vi "coord.vi"(7 "error in":errorcluster) -> (27 "error out":errorcluster)   [LabVIEW 2019]
uses:
  <vilib>/vision/Pattern Matching.llb/IMAQ Pattern Match Advanced Options.ctl
  <vilib>/vision/NI_Vision_Development_Module.lvlib
panel:
  in  "selected path":path
  out "ROI Descriptor out":T1 {"Contours"."Type" items=["No Selection", "Point", "Line", "Rectangle", "Oval", "Polygon", "Freehand Region", "Annulus", "Unused2", "Unused3", "Broken Line", "Freehand Line", "Rotated Rectangle"]}
  out "Image Out":T2(plugin-control)
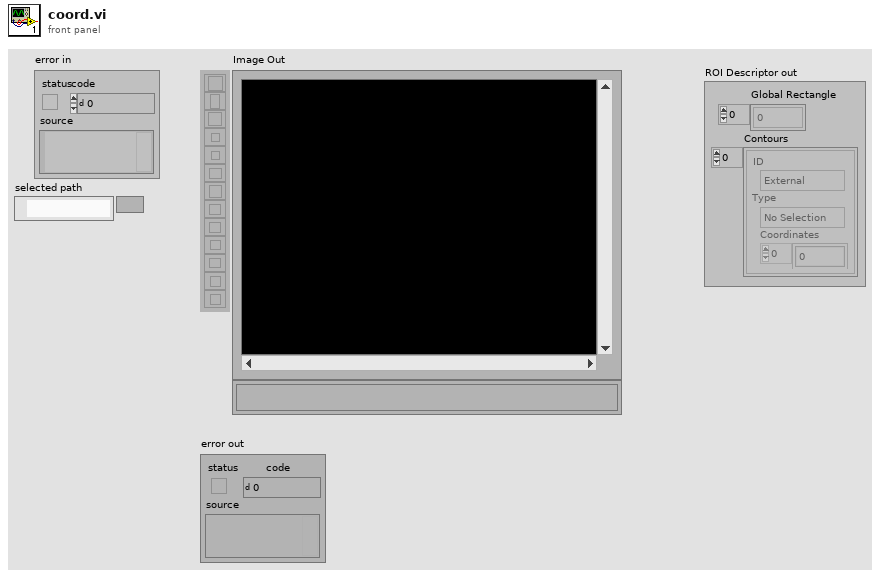
[diagram p1: front panel]
types:
  T1 = typedef "ROI Descriptor" = cluster{"Global Rectangle":i32[], "Contours":cluster{"ID":enum32{"External", "Internal"}, "Type":u32, "Coordinates":i32[]}[]}
  T2 = typedef "IMAQ Image.ctl" = refnum<image>
  T3 = cluster{"Global Rectangle":i32[], "Contours":cluster{"ID":enum32{"External", "Internal"}, "Type":u32, "Coordinates":i32[]}[]}
  T4 = cluster{"Origin":cluster{"X":sgl, "Y":sgl}, "Angle (deg)":sgl, "Axis Reference":u32}
  T5 = enum16{"Reset", "Update Coordinate System", "Get Coordinate System"}
  T6 = enum16{"Horizontal Motion", "Vertical Motion", "Horizontal and Vertical Motion", "Horizontal, Vertical and Angular Motion"}
  T7 = typedef "IMAQ Pattern Match Advanced Options.ctl" = u16
  T8 = cluster{"Number of Matches Requested":i32, "Minimum Match Score":sgl, "Angle Ranges":cluster{"Start Angle":sgl, "End Angle":sgl}[]}
  T9 = typedef "Image Type" = u32
  T10 = cluster{"Position":cluster{"x":sgl, "y":sgl}, "Angle":sgl, "Scale":sgl, "Score":sgl, "Bounding Box":cluster{"x":sgl, "y":sgl}[]}[]
  T11 = typedef "IMAQ Coordinate System" = cluster{"Reference System":cluster{"Origin":cluster{"X":sgl, "Y":sgl}, "Angle (deg)":sgl, "Axis Reference":u32}, "Measurement System":cluster{"Origin":cluster{"X":sgl, "Y":sgl}, "Angle (deg)":sgl, "Axis Reference":u32}}
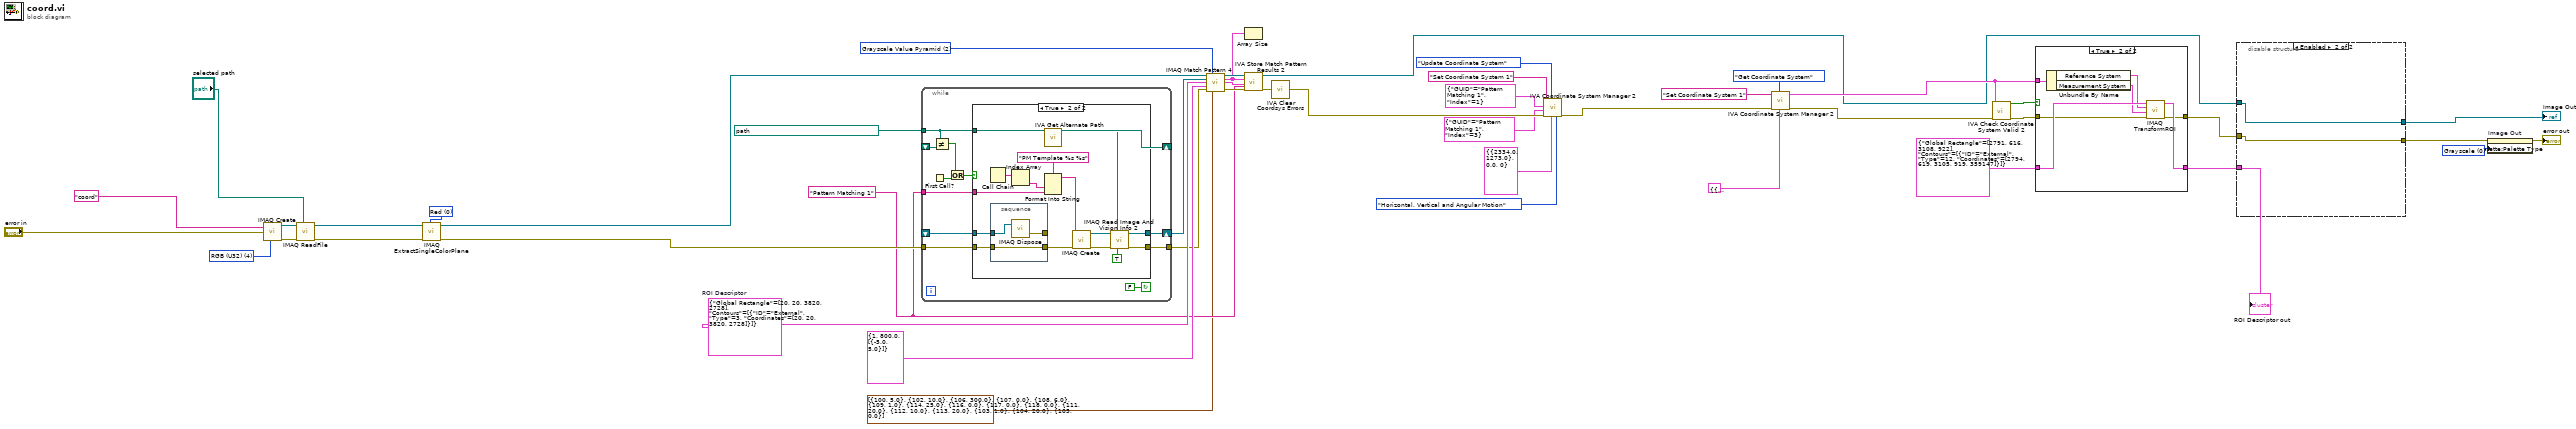
[diagram p0: block diagram]
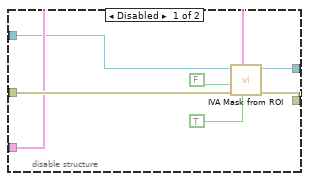
[diagram p2: hidden frame]
diagram:
  w3 = u32 0 items=["Grayscale", "Binary", "Gradient", "Rainbow", "Temperature", "User Defined", "Binary 16 Bit", "Gradient 16 Bit", "Rainbow 16 Bit", "Temperature 16 Bit", "User Defined 16 Bit"] ("Palette Type")
  w35 = 2 items=["All", "Low Discrepancy Sampling", "Grayscale Value Pyramid", "Gradients Pyramid"] ("Algorithm")
  w32 = "Pattern Matching 1" ("Step Name")
  w34 = T3 {"Global Rectangle"=[20, 20, 3820, 2728], "Contours"=[{"ID"=enum."External", "Type"=3, "Coordinates"=[20, 20, 3820, 2728]}]}  # ROI Descriptor
  w42 = 0 items=["Red", "Green", "Blue", "Hue", "Saturation", "Luminance", "Value", "Intensity"] ("Color Plane")
  w43 = T9 4 items=["Grayscale (U8)", "Grayscale (I16)", "Grayscale (SGL)", "Complex (CSG)", "RGB (U32)", "HSL (U32)", "RGB (U64)", "Grayscale (U16)"] ("Image Type")
  n1 = call "IMAQ Create"("Image Name"="coord", "Image Type"=w43, "error in (no error)"="error in") -> ("New Image"=w46:T2, "error out"=w45:errorcluster)  [unwired: 1 in, 1 out]
  n2 = call "IMAQ ReadFile"("File Path"="selected path", "error in (no error)"=w45, "Image"=w46) -> ("error out"=w47:errorcluster, "Image Out"=w41:T2)  [unwired: 2 in, 5 out]
  n3 = call "IMAQ ExtractSingleColorPlane"("Color Plane"=w42, "error in (no error)"=w47, "Image Src"=w41) -> ("error out"=w40:errorcluster, "Image Dst Out"=w38:T2)  [unwired: 1 in, 6 out]
  n4 = while {
    shift-right: [w58] -> w29
    shift-left: _ -> [w57]
    tunnel: [w55] -> w28
    tunnel: w40 -> [w54]
    tunnel: path "D:/vicomm case/為生 AI/AI Picture/11.png" ("Template File Path") -> [w51]
    tunnel: w32 -> [w53]
    shift-right: [w51] -> _
    shift-left: _ -> [w52]
    stop <- FALSE continue-if-true
    n5 = First Call?() -> (First Call?: T/F=w50:bool)
    n6 = Not Equal?(x=w51, y=w52) -> (x != y?=w49:bool)
    n7 = Or(x=w49, y=w50) -> (x .or. y?=w48:bool)
    n8 = case shown="True" w48 {
      tunnel: [w60 w65] -> w58
      tunnel: w57 -> [w60 w69]
      tunnel: [w59 w66] -> w55
      tunnel: w54 -> [w59 w68]
      tunnel: w51 -> [_ w70]
      tunnel: w53 -> [_ w71]
      frame False {
      }
      frame True {
        n9 = Call Chain() -> (call chain=w73:string[])
        n10 = stacked-sequence {
          tunnel: w69 -> [w78]
          tunnel: w68 -> [w77]
          tunnel: [w77] -> w62
          tunnel: [w76] -> _
          frame #0 {
            n11 = call "IMAQ Dispose"("Image"=w78) -> ("error out"=w76:errorcluster)  [unwired: 2 in, 3 out]
          }
        }
        n12 = Index Array(array=w73) -> (element=w72:string)  [unwired: 1 in]
        n13 = call <vilib>:"IVA Get Alternate Path.vi"("Path In"=w70) -> ("Path Out"=w67:path)  [unwired: 10 out]
        n14 = Format Into String(format string="PM Template %s %s" ("Image Name"), w72, w71) -> (resulting string=w75:string)  [unwired: 2 in, 1 out]
        n15 = call "IMAQ Create"("Image Name"=w75, "error in (no error)"=w62) -> ("New Image"=w64:T2, "error out"=w63:errorcluster)  [unwired: 2 in, 1 out]
        n16 = call "IMAQ Read Image And Vision Info 2"("Use File Path Image Type"=TRUE, "File Path"=w67, "error in (no error)"=w63, "Image"=w64) -> ("error out"=w66:errorcluster, "Image Out"=w65:T2)  [unwired: 5 in, 1 out]
      }
    }
  }
  n17 = call "IMAQ Match Pattern 4"("Image"=w38, "Algorithm"=w35, "Template Image"=w29, "ROI Descriptor"=w34, "Parameters"=T8 {"Number of Matches Requested"=1, "Minimum Match Score"=800.0, "Angle Ranges"=[{"Start Angle"=-5.0, "End Angle"=5.0}]}, "error in (no error)"=w28, "Advanced Options"=cluster{"Item":T7, "Value":dbl}[] [{"Item"=100, "Value"=5.0}, {"Item"=102, "Value"=10.0}, {"Item"=106, "Value"=300.0}, {"Item"=107, "Value"=0.0}, {"Item"=108, "Value"=6.0}, {"Item"=109, "Value"=1.0}, {"Item"=114, "Value"=25.0}, {"Item"=116, "Value"=0.0}, {"Item"=117, "Value"=0.0}, {"Item"=118, "Value"=0.0}, {"Item"=111, "Value"=20.0}, {"Item"=112, "Value"=10.0}, {"Item"=113, "Value"=20.0}, {"Item"=103, "Value"=1.0}, {"Item"=104, "Value"=20.0}, {"Item"=105, "Value"=0.0}]) -> ("Image (duplicate)"=w36:T2, "Matches (pixel)"=w31:T10, "Matches (real-world)"=w30:T10, "error out"=w37:errorcluster)  [unwired: 4 in, 1 out]
  n18 = Array Size(array=w31) -> ()  [unwired: 1 out]
  n19 = call <vilib>:"IVA Store Match Pattern Results 2.vi"("Step Name"=w32, "error in (no error)"=w37, "Matches (real-world)"=w30, "Matches (pixel)"=w31, "Image in"=w36) -> ("error out"=w27:errorcluster, "Image dup"=w7:T2)  [unwired: 1 in, 4 out]
  n20 = call <vilib>:"IVA Clear Coordsys Errors.vi"("error in (no error)"=w27) -> ("error out"=w26:errorcluster)  [unwired: 10 in]
  n21 = call <vilib>:"IVA Coordinate System Manager 2.vi"("Mode"=T6."Horizontal, Vertical and Angular Motion", "Reference System"=T4 {"Origin"={"X"=2334.0, "Y"=1273.0}, "Angle (deg)"=0.0, "Axis Reference"=0}, "Function"=T5."Update Coordinate System", "error in (no error)"=w26, "Angle ID"=cluster{"GUID":string, "Index":i32} {"GUID"="Pattern Matching 1", "Index"=3}, "Origin ID"=cluster{"GUID":string, "Index":i32} {"GUID"="Pattern Matching 1", "Index"=1}, "Coordinate System Name"="Set Coordinate System 1") -> ("error out"=w18:errorcluster)  [unwired: 4 out]
  n22 = call <vilib>:"IVA Coordinate System Manager 2.vi"("Reference System"=T4 {"Origin"={"X"=2352.643, "Y"=1231.139}, "Angle (deg)"=359.1477, "Axis Reference"=0}, "Function"=T5."Get Coordinate System", "error in (no error)"=w18, "Coordinate System Name"="Set Coordinate System 1") -> ("error out"=w15:errorcluster, "Coordinate System Out"=w11:T11)  [unwired: 3 in, 3 out]
  n23 = call <vilib>:"IVA Check Coordinate System Valid 2.vi"("error in (no error)"=w15, "Coordinate System"=w11) -> ("error out"=w9:errorcluster, "Valid?"=w10:bool)  [unwired: 8 out]
  n24 = case shown="True" w10 {
    tunnel: T3 {"Global Rectangle"=[2791, 616, 3108, 922], "Contours"=[{"ID"=enum."External", "Type"=12, "Coordinates"=[2794, 619, 3105, 919, 359147]}]} ("ROI Descriptor") -> [w80 w87]
    tunnel: [w80 w84] -> w8
    tunnel: [w79 w83] -> w12
    tunnel: w11 -> [_ w82]
    tunnel: w9 -> [w79 w81]
    frame False {
    }
    frame True {
      n25 = Unbundle By Name(w82) -> ("Reference System"=w86:T4, "Measurement System"=w85:T4)
      n26 = call "IMAQ TransformROI"("error in (no error)"=w81, "New Reference"=w85, "Base Reference"=w86, "ROI Descriptor"=w87) -> ("error out"=w83:errorcluster, "ROI Descriptor out"=w84:T1)  [unwired: 6 out]
    }
  }
  "ROI Descriptor out" <- w8
  n27 = disable-structure shown="Enabled" {
    disable-tunnel: w12 -> [w94 w96]
    disable-tunnel: w8 -> [w93 _]
    disable-tunnel: w7 -> [w91 w95]
    disable-tunnel: [w89 w96] -> w6
    disable-tunnel: [w88 w95] -> w4
    frame Disabled {
      n28 = call <vilib>:"IVA Mask from ROI.vi"("Shrink"=TRUE, "ROI Descriptor"=w93, "error in (no error)"=w94, "Out / In"=FALSE, "Image Src"=w91) -> ("error out"=w89:errorcluster, "Image Out"=w88:T2)  [unwired: 5 out]
    }
    frame Enabled {
    }
  }
  "Image Out" <- w4
  n29 = property on="Image Out" class="ImageControl"(error in=w6, "Palette:Palette Type"=w3) -> (error out=→"error out":errorcluster)  [unwired: 1 in, 1 out]
